vi "construct.vi"(8 "error in (no error)":errorcluster, 11 "CompactDAQ in":refnum<class "CompactDAQ.lvclass">) -> (0 "error out":errorcluster, 3 "CompactDAQ out":refnum<class "CompactDAQ.lvclass">)   [LabVIEW 2017, in "CompactDAQ.lvclass"]
uses:
  CompactDAQ.lvclass
  Configuration/CompactDAQ Configuration.lvclass
  \\Mac\Home/Documents/MAL-Framework/user.lib/Common Components/Hardware/HW Config/HW Configuration.lvclass
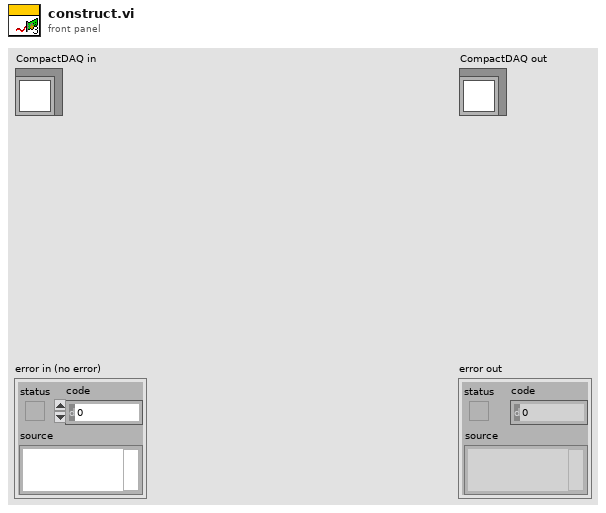
[diagram p1: front panel]
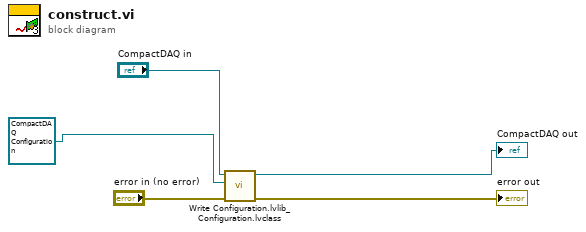
[diagram p0: block diagram]
diagram:
  n1 = call-dynamic "Write Configuration.lvlib_Configuration.lvclass.vi"("error in (no error)"="error in (no error)", "Hardware.lvlib:HW Configuration.lvclass"=refnum<class "CompactDAQ Configuration.lvclass"> refnum ("CompactDAQ Configuration.lvclass"), "CompactDAQ in"="CompactDAQ in") -> ("error out"=→"error out":errorcluster, "CompactDAQ out"=→"CompactDAQ out":refnum<class "CompactDAQ.lvclass">)  [unwired: 7 in]
